vi "SMSD_powerstep01_cmd.vi"(8 "error in (no error)":errorcluster, 9 "DATA (0)":u32 format="%x", 10 "COMMAND (END)":T1(ring), 11 "SMSD in":refnum<class "SMSD.lvclass">) -> (0 "error out":errorcluster, 1 "timed out?":bool, 2 "data":u8[](array[numeric]), 3 "SMSD out":refnum<class "SMSD.lvclass">)   [LabVIEW 2019, in "SMSD.lvclass"]
uses:
  SMSD.lvclass
  C:/my_projects/projects/Algorithms/Labview/19/Modbus/MB_TCP2/MB_TCP.lvclass
  SMSD.lvclass/SMSD.ctl
  MB_TCP.lvclass/MB_TCP.ctl
  NI_modbus_upd/TCP/TCP.lvclass/TCP.ctl
  SMSD_LAN_COMMAND.vi
  <vilib>/Utility/error.llb/Clear Errors.vi
  NI_modbus_upd/TCP/TCP.lvclass
  MB_TCP.lvclass
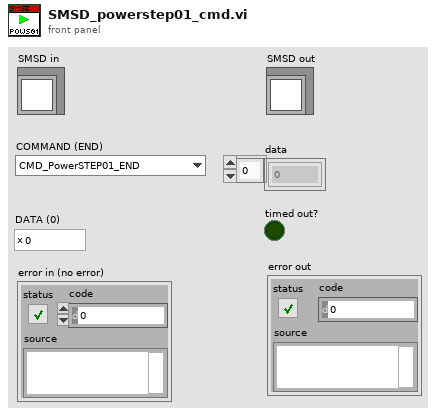
[diagram p1: front panel]
types:
  T1 = enum8{"CMD_PowerSTEP01_END", "CMD_PowerSTEP01_GET_SPEED", "CMD_PowerSTEP01_STATUS_IN_EVENT", "CMD_PowerSTEP01_SET_MODE", "CMD_PowerSTEP01_GET_MODE", "CMD_PowerSTEP01_SET_MIN_SPEED", "CMD_PowerSTEP01_SET_MAX_SPEED", "CMD_PowerSTEP01_SET_ACC", "CMD_PowerSTEP01_SET_DEC", "CMD_PowerSTEP01_SET_FS_SPEED", "CMD_PowerSTEP01_SET_MASK_EVENT", "CMD_PowerSTEP01_GET_ABS_POS", "CMD_PowerSTEP01_GET_EL_POS", "CMD_PowerSTEP01_GET_STATUS_AND_CLR", "CMD_PowerSTEP01_RUN_F", "CMD_PowerSTEP01_RUN_R", "CMD_PowerSTEP01_MOVE_F", "CMD_PowerSTEP01_MOVE_R", "CMD_PowerSTEP01_GO_TO_F", "CMD_PowerSTEP01_GO_TO_R", "CMD_PowerSTEP01_GO_UNTIL_F", "CMD_PowerSTEP01_GO_UNTIL_R", "CMD_PowerSTEP01_SCAN_ZERO_F", "CMD_PowerSTEP01_SCAN_ZERO_R", "CMD_PowerSTEP01_SCAN_LABEL_F", "CMD_PowerSTEP01_SCAN_LABEL_R", "CMD_PowerSTEP01_GO_ZERO", "CMD_PowerSTEP01_GO_LABEL", "CMD_PowerSTEP01_GO_TO", "CMD_PowerSTEP01_RESET_POS", "CMD_PowerSTEP01_RESET_POWERSTEP01", "CMD_PowerSTEP01_SOFT_STOP", "CMD_PowerSTEP01_HARD_STOP", "CMD_PowerSTEP01_SOFT_HI_Z", "CMD_PowerSTEP01_HARD_HI_Z", "CMD_PowerSTEP01_SET_WAIT", "CMD_PowerSTEP01_SET_RELE", "CMD_PowerSTEP01_CLR_RELE", "CMD_PowerSTEP01_GET_RELE", "CMD_PowerSTEP01_WAIT_IN0", "CMD_PowerSTEP01_WAIT_IN1", "CMD_PowerSTEP01_GOTO_PROGRAM", "CMD_PowerSTEP01_GOTO_PROGRAM_IF_IN0", "CMD_PowerSTEP01_GOTO_PROGRAM_IF_IN1", "CMD_PowerSTEP01_LOOP_PROGRAM", "CMD_PowerSTEP01_CALL_PROGRAM", "CMD_PowerSTEP01_RETURN_PROGRAM", "CMD_PowerSTEP01_START_PROGRAM_MEM0", "CMD_PowerSTEP01_START_PROGRAM_MEM1", "CMD_PowerSTEP01_START_PROGRAM_MEM2", "CMD_PowerSTEP01_START_PROGRAM_MEM3", "CMD_PowerSTEP01_STOP_PROGRAM_MEM", "CMD_PowerSTEP01_STEP_CLOCK", "CMD_PowerSTEP01_STOP_USB", "CMD_PowerSTEP01_GET_MIN_SPEED", "CMD_PowerSTEP01_GET_MAX_SPEED", "CMD_PowerSTEP01_GET_STACK", "CMD_PowerSTEP01_GOTO_PROGRAM_IF_ZERO", "CMD_PowerSTEP01_GOTO_PROGRAM_IF_IN_ZERO", "CMD_PowerSTEP01_WAIT_CONTINUE", "CMD_PowerSTEP01_SET_WAIT_2", "CMD_PowerSTEP01_SCAN_MARK2_F", "CMD_PowerSTEP01_SCAN_MARK2_R"}
  T2 = enum8{"CODE_CMD_REQUEST", "CODE_CMD_RESPONSE", "CODE_CMD_POWERSTEP01", "CODE_CMD_POWERSTEP01_W_MEM0", "CODE_CMD_POWERSTEP01_W_MEM1", "CODE_CMD_POWERSTEP01_W_MEM2", "CODE_CMD_POWERSTEP01_W_MEM3", "CODE_CMD_POWERSTEP01_R_MEM0", "CODE_CMD_POWERSTEP01_R_MEM1", "CODE_CMD_POWERSTEP01_R_MEM2", "CODE_CMD_POWERSTEP01_R_MEM3", "CODE_CMD_CONFIG_SET", "CODE_CMD_CONFIG_GET", "CODE_CMD_PASSWORD_SET", "CODE_CMD_ERROR_GET"}
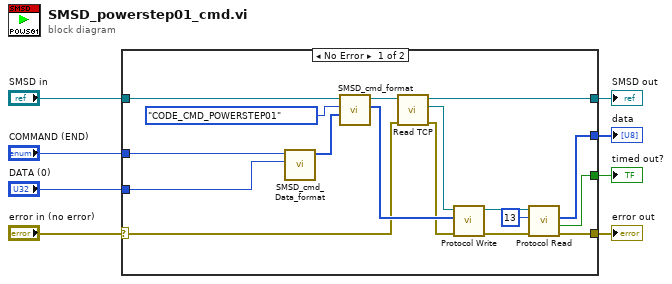
[diagram p0: block diagram]
diagram:
  n1 = case shown="No Error" "error in (no error)" {
    selector: "error in (no error)" -> [w10 w27]
    tunnel: [w25 _] -> w8
    tunnel: [w24 w27] -> w7
    tunnel: "COMMAND (END)" -> [w23 _]
    tunnel: "SMSD in" -> [w16 w26]
    tunnel: [w12 w26] -> w4
    tunnel: "DATA (0)" -> [w15 _]
    tunnel: [w14 _] -> w1
    frame No Error {
      n2 = call "SMSD_cmd_Data_format.vi"("DATA (0)"=w15, "COMMAND (END)"=w23) -> ("SMSD_CMD_out"=w22:u8[])  [unwired: 9 in]
      n3 = call "SMSD_cmd_format.vi"("DATA"=w22, "CMD_TYPE"=T2."CODE_CMD_POWERSTEP01", "SMSD in"=w16) -> ("LAN_CMD_out"=w18:u8[], "SMSD out"=w13:refnum<class "SMSD.lvclass">)  [unwired: 7 in]
      n4 = call "Read TCP.vi"("error in (no error)"=w10, "MB_TCP in"=w13) -> ("error out"=w9:errorcluster, "TCP"=w11:refnum<class "TCP.lvclass">, "MB_TCP out"=w12:refnum<class "SMSD.lvclass">)  [unwired: 7 in]
      n5 = call "Protocol Write.vi"("error in (no error)"=w9, "data"=w18, "protocol layer in"=w11) -> ("error out"=w21:errorcluster, "protocol layer out"=w20:refnum<class "TCP.lvclass">)  [unwired: 6 in, 1 out]
      n6 = call "Protocol Read.vi"("error in (no error)"=w21, "bytes to read"=13, "TCP in"=w20) -> ("error out"=w24:errorcluster, "timed out?"=w14:bool, "data"=w25:u8[])  [unwired: 5 in, 1 out]
    }
    frame Error {
    }
  }
  "data" <- w8
  "error out" <- w7
  "SMSD out" <- w4
  "timed out?" <- w1
